vi "zadanie_3.vi"() -> ()   [LabVIEW 2020]
panel:
  in  "pierwszy wyraz":dbl
  in  "zadane n":dbl
  out "suma":dbl
  in  "stop":bool
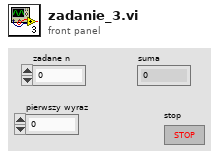
[diagram p1: front panel]
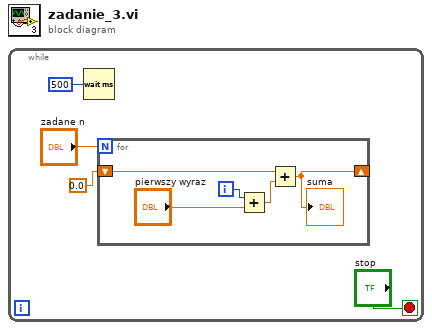
[diagram p0: block diagram]
diagram:
  n1 = while {
    stop <- "stop" stop-if-true
    n2 = Wait (ms)(milliseconds to wait=500) -> ()  [unwired: 1 out]
    n3 = for {
      N: "zadane n" -> [_]
      shift-right: [w8] -> _
      shift-left: 0.0 -> [w9]
      i -> [w6]
      n4 = Add(x=w6, y="pierwszy wyraz") -> (x+y=w7:dbl)
      n5 = Add(x=w9, y=w7) -> (x+y=w8:dbl)
      "suma" <- w8
    }
  }
